vi "Read failTPDOCounter.vi"(8 "error in (no error)":errorcluster, 11 "Orion_BMS in":refnum<class "Orion_BMS.lvclass">) -> (0 "error out":errorcluster, 2 "failTPDOCounter":u32, 3 "Orion_BMS out":refnum<class "Orion_BMS.lvclass">)   [LabVIEW 2017, in "Orion_BMS.lvclass"]
uses:
  Orion_BMS.lvclass
  Orion_BMS.lvclass/Orion_BMS.ctl
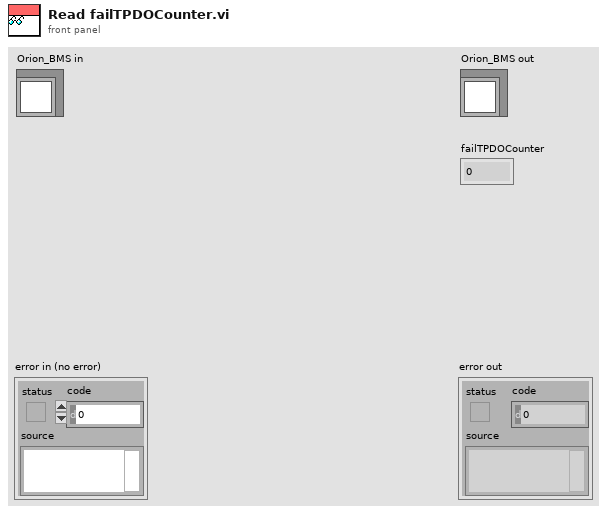
[diagram p1: front panel]
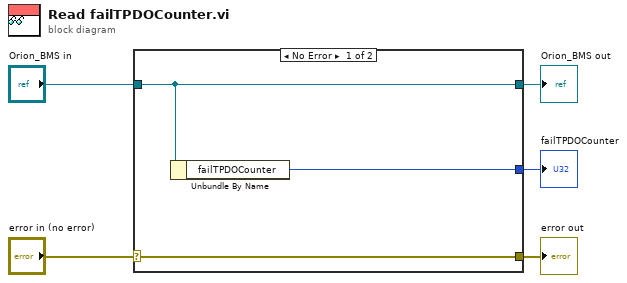
[diagram p0: block diagram]
diagram:
  n1 = case shown="No Error" "error in (no error)" {
    selector: "error in (no error)" -> [w8 w9]
    tunnel: [w8 w9] -> w4
    tunnel: [w7 w10] -> w2
    tunnel: "Orion_BMS in" -> [w7 w10]
    tunnel: [w6 _] -> w1
    frame No Error {
      n2 = Unbundle By Name(w7) -> ("failTPDOCounter"=w6:u32)
    }
    frame Error {
    }
  }
  "error out" <- w4
  "Orion_BMS out" <- w2
  "failTPDOCounter" <- w1
